vi "svm_train.vi"(8 "error in (no error)":errorcluster, 10 "Parameters":T2, 11 "Problem":T6) -> (0 "error out":errorcluster, 3 "Model":T1)   [LabVIEW 2015]
uses:
  Controls/svm_problem.ctl
  Controls/svm_node.ctl
  Controls/svm_parameter.ctl
  Controls/svm_type.ctl
  Controls/svm_kernel_type.ctl
  Controls/svm_model.ctl
  Controls/svm_node_padded.ctl
  Controls/svm_model_padded.ctl
  bin/x64/LabVIEW-libsvm.dll
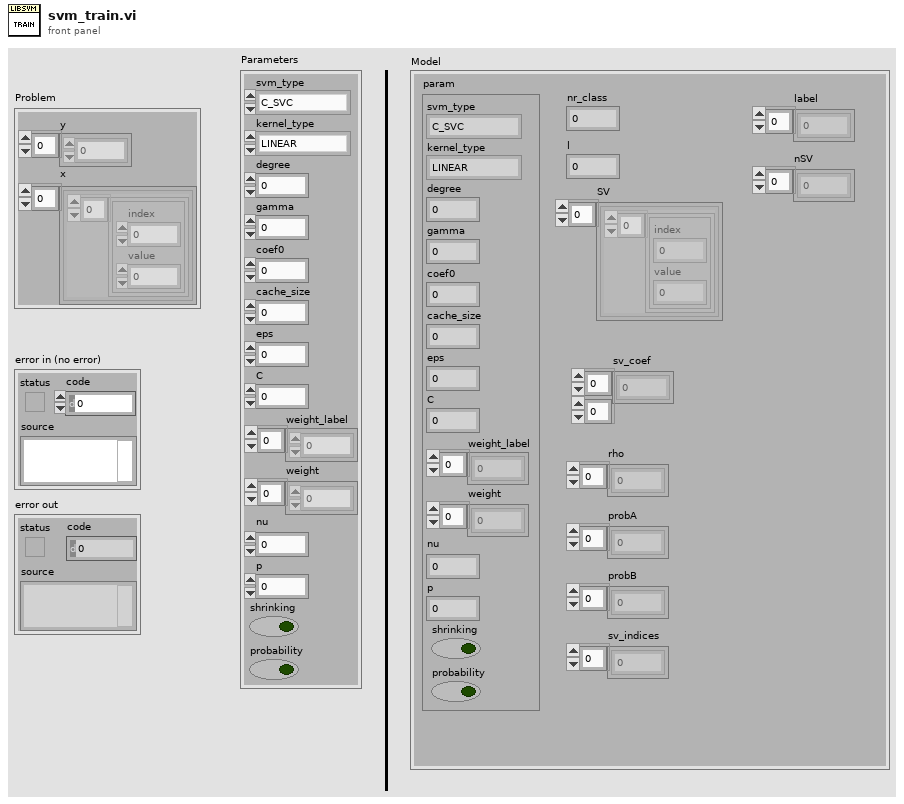
[diagram p1: front panel]
types:
  T1 = typedef "svm_model.ctl" = cluster{"param":T2, "nr_class":i32, "l":i32, "SV":cluster{"Array":T5[]}[], "sv_coef":dbl[][], "rho":dbl[], "probA":dbl[], "probB":dbl[], "sv_indices":i32[], "label":i32[], "nSV":i32[]}
  T2 = typedef "svm_parameter.ctl" = cluster{"svm_type":T3, "kernel_type":T4, "degree":i32, "gamma":dbl, "coef0":dbl, "cache_size":dbl, "eps":dbl, "C":dbl, "weight_label":i32[], "weight":dbl[], "nu":dbl, "p":dbl, "shrinking":bool, "probability":bool}
  T3 = typedef "svm_type.ctl" = enum32{"C_SVC", "NU_SVC", "ONE_CLASS", "EPSILON_SVR", "NU_SVR"}
  T4 = typedef "svm_kernel_type.ctl" = enum32{"LINEAR", "POLY", "RBF", "SIGMOID", "PRECOMPUTED"}
  T5 = typedef "svm_node.ctl" = cluster{"index":i32, "value":dbl}
  T6 = typedef "svm_problem.ctl" = cluster{"y":dbl[], "x":cluster{T5[]}[]}
  T7 = typedef "svm_model_padded.ctl" = cluster{"param":T2, "nr_class":i32, "l":i32, "SV":cluster{"Array":T8[]}[], "sv_coef":dbl[][], "rho":dbl[], "probA":dbl[], "probB":dbl[], "sv_indices":i32[], "label":i32[], "nSV":i32[]}
  T8 = typedef "svm_node_padded.ctl" = cluster{"index":i32, "padding":i32, "value":dbl}
  T9 = typedef "svm_problem_padded.ctl" = cluster{"y":dbl[], "x":cluster{T8[]}[]}
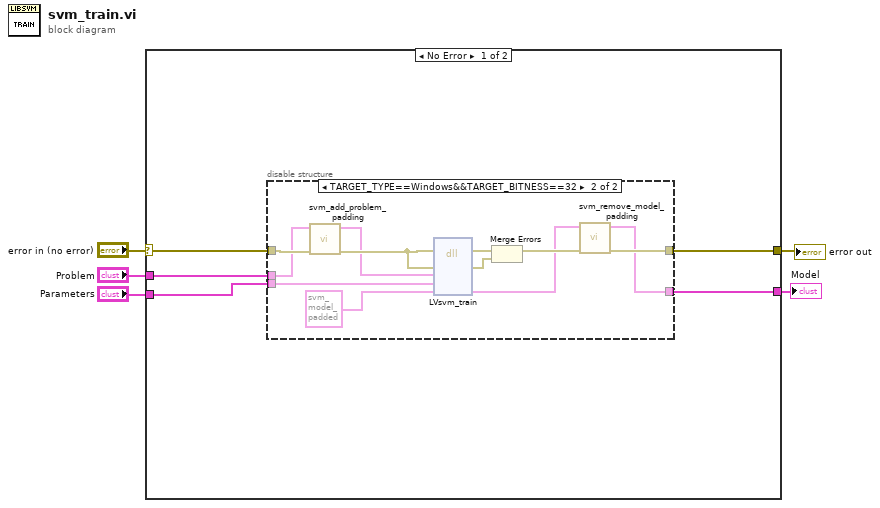
[diagram p0: block diagram]
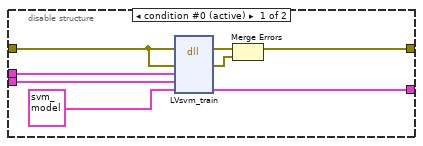
[diagram p2: hidden frame]
diagram:
  n1 = case shown="No Error" "error in (no error)" {
    selector: "error in (no error)" -> [w10 w31]
    tunnel: [w9 w31] -> w5
    tunnel: "Problem" -> [w8 _]
    tunnel: "Parameters" -> [w7 _]
    tunnel: [w6 _] -> w1
    frame No Error {
      n2 = disable-structure shown="TARGET_TYPE==Windows&&TARGET_BITNESS==32" {
        disable-tunnel: w10 -> [w18 w27]
        disable-tunnel: [w15 w22] -> w9
        disable-tunnel: w8 -> [w14 w25]
        disable-tunnel: [w13 w20] -> w6
        disable-tunnel: w7 -> [w12 w28]
        frame condition #0 (active) {
          n3 = dll-call lib="C:/dev/LabVIEW-libsvm/LabVIEW/bin/x64/LabVIEW-libsvm.dll" fn="LVsvm_train"(error in=w18, "lvErr"=w18, "prob_in"=w14, "param_in"=w12, "model_out"=T1 {"param"={"svm_type"=enum."C_SVC", "kernel_type"=enum."LINEAR", "degree"=0, "gamma"=0.0, "coef0"=0.0, "cache_size"=0.0, "eps"=0.0, "C"=0.0, "weight_label"=[], "weight"=[], "nu"=0.0, "p"=0.0, "shrinking"=FALSE, "probability"=FALSE}, "nr_class"=0, "l"=0, "SV"=[], "sv_coef"=[], "rho"=[], "probA"=[], "probB"=[], "sv_indices"=[], "label"=[], "nSV"=[]} ("svm_model")) -> (error out=w17:errorcluster, "lvErr"=w16:errorcluster, "model_out"=w13:T1)  [unwired: 5 in, 1 out]
          n4 = Merge Errors(w17, w16) -> (w15:errorcluster)
        }
        frame condition #1 {
          n5 = call "svm_add_problem_padding.vi"("error in (no error)"=w27, "problem"=w25) -> ("error out"=w26:errorcluster, "padded problem"=w24:T9)  [unwired: 8 in]
          n6 = dll-call lib="C:/dev/LabVIEW-libsvm/LabVIEW/bin/x64/LabVIEW-libsvm.dll" fn="LVsvm_train"(error in=w26, "lvErr"=w26, "prob_in"=w24, "param_in"=w28, "model_out"=T7 {"param"={"svm_type"=enum."C_SVC", "kernel_type"=enum."LINEAR", "degree"=0, "gamma"=0.0, "coef0"=0.0, "cache_size"=0.0, "eps"=0.0, "C"=0.0, "weight_label"=[], "weight"=[], "nu"=0.0, "p"=0.0, "shrinking"=FALSE, "probability"=FALSE}, "nr_class"=0, "l"=0, "SV"=[], "sv_coef"=[], "rho"=[], "probA"=[], "probB"=[], "sv_indices"=[], "label"=[], "nSV"=[]} ("svm_model")) -> (error out=w30:errorcluster, "lvErr"=w29:errorcluster, "model_out"=w21:T7)  [unwired: 5 in, 1 out]
          n7 = Merge Errors(w30, w29) -> (w23:errorcluster)
          n8 = call "svm_remove_model_padding.vi"("error in (no error)"=w23, "Padded model"=w21) -> ("error out"=w22:errorcluster, "Model"=w20:T1)  [unwired: 8 in]
        }
      }
    }
    frame Error {
    }
  }
  "error out" <- w5
  "Model" <- w1
